vi "Filter_of_Tracks_based_on_areas_differences-2.vi"(4 "error IN":errorcluster, 5 "[IN] Movie Values":T2 {"Particle Fil Setups"."Type of particle filter"."Measurement Parameter" items=["Center of Mass X", "Center of Mass Y", "First Pixel X", "First Pixel Y", "Bounding Rect Left", "Bounding Rect Top", "Bounding Rect Right", "Bounding Rect Bottom", "Max Feret Diameter Start X", "Max Feret Diameter Start Y", "Max Feret Diameter End X", "Max Feret Diameter End Y", "Max Horiz. Segment Length Left", "Max Horiz. Segment Length Right", "Max Horiz. Segment Length Row", "-", "Bounding Rect Width", "Bounding Rect Height", "Bounding Rect Diagonal", "Perimeter", "Convex Hull Perimeter", "Holes' Perimeter", "Max Feret Diameter", "Equivalent Ellipse Major Axis", "Equivalent Ellipse Minor Axis", "Equivalent Ellipse Minor Axis (Feret)", "Equivalent Rect Long Side", "Equivalent Rect Short Side", "Equivalent Rect Diagonal", "Equivalent Rect Short Side (Feret)", "Average Horiz. Segment Length", "Average Vert. Segment Length", "Hydraulic Radius", "Waddel Disk Diameter", "-", "Area", "Holes' Area", "Particle & Holes' Area", "Convex Hull Area", "Image Area", "-", "Number of Holes", "Number of Horiz. Segments", "Number of Vert. Segments", "-", "Orientation", "Max Feret Diameter Orientation", "-", "% Area/Image Area", "% Area/(Particle & Holes' Area)", "Ratio of Equivalent Ellipse Axes", "Ratio of Equivalent Rect Sides", "-", "Elongation Factor", "Compactness Factor", "Heywood Circularity Factor", "Type Factor", "-", "Sum X", "Sum Y", "Sum XX", "Sum XY", "Sum YY", "Sum XXX", "Sum XXY", "Sum XYY", "Sum YYY", "-", "Moment of Inertia XX", "Moment of Inertia XY", "Moment of Inertia YY", "Moment of Inertia XXX", "Moment of Inertia XXY", "Moment of Inertia XYY", "Moment of Inertia YYY", "Norm. Moment of Inertia XX", "Norm. Moment of Inertia XY", "Norm. Moment of Inertia YY", "Norm. Moment of Inertia XXX", "Norm. Moment of Inertia XXY", "Norm. Moment of Inertia XYY", "Norm. Moment of Inertia YYY", "Hu Moment 1", "Hu Moment 2", "Hu Moment 3", "Hu Moment 4", "Hu Moment 5", "Hu Moment 6", "Hu Moment 7"]}, 6 "[IN] Part of mean value (amplitude)\nFor making filtering criteria":dbl, 7 "[IN] Tracks w/t Problems":T3(array[cluster])) -> (0 "error OUT":errorcluster, 2 "[OUT] Oscillating Tracks":cluster{"Short Tracks":dbl[], "Start Pos":i32}[](array[cluster]), 3 "[OUT] Stable Tracks (Filtered)":T3(array[cluster]))   [LabVIEW 2013]
uses:
  <vilib>/Analysis/NI_AALBase.lvlib
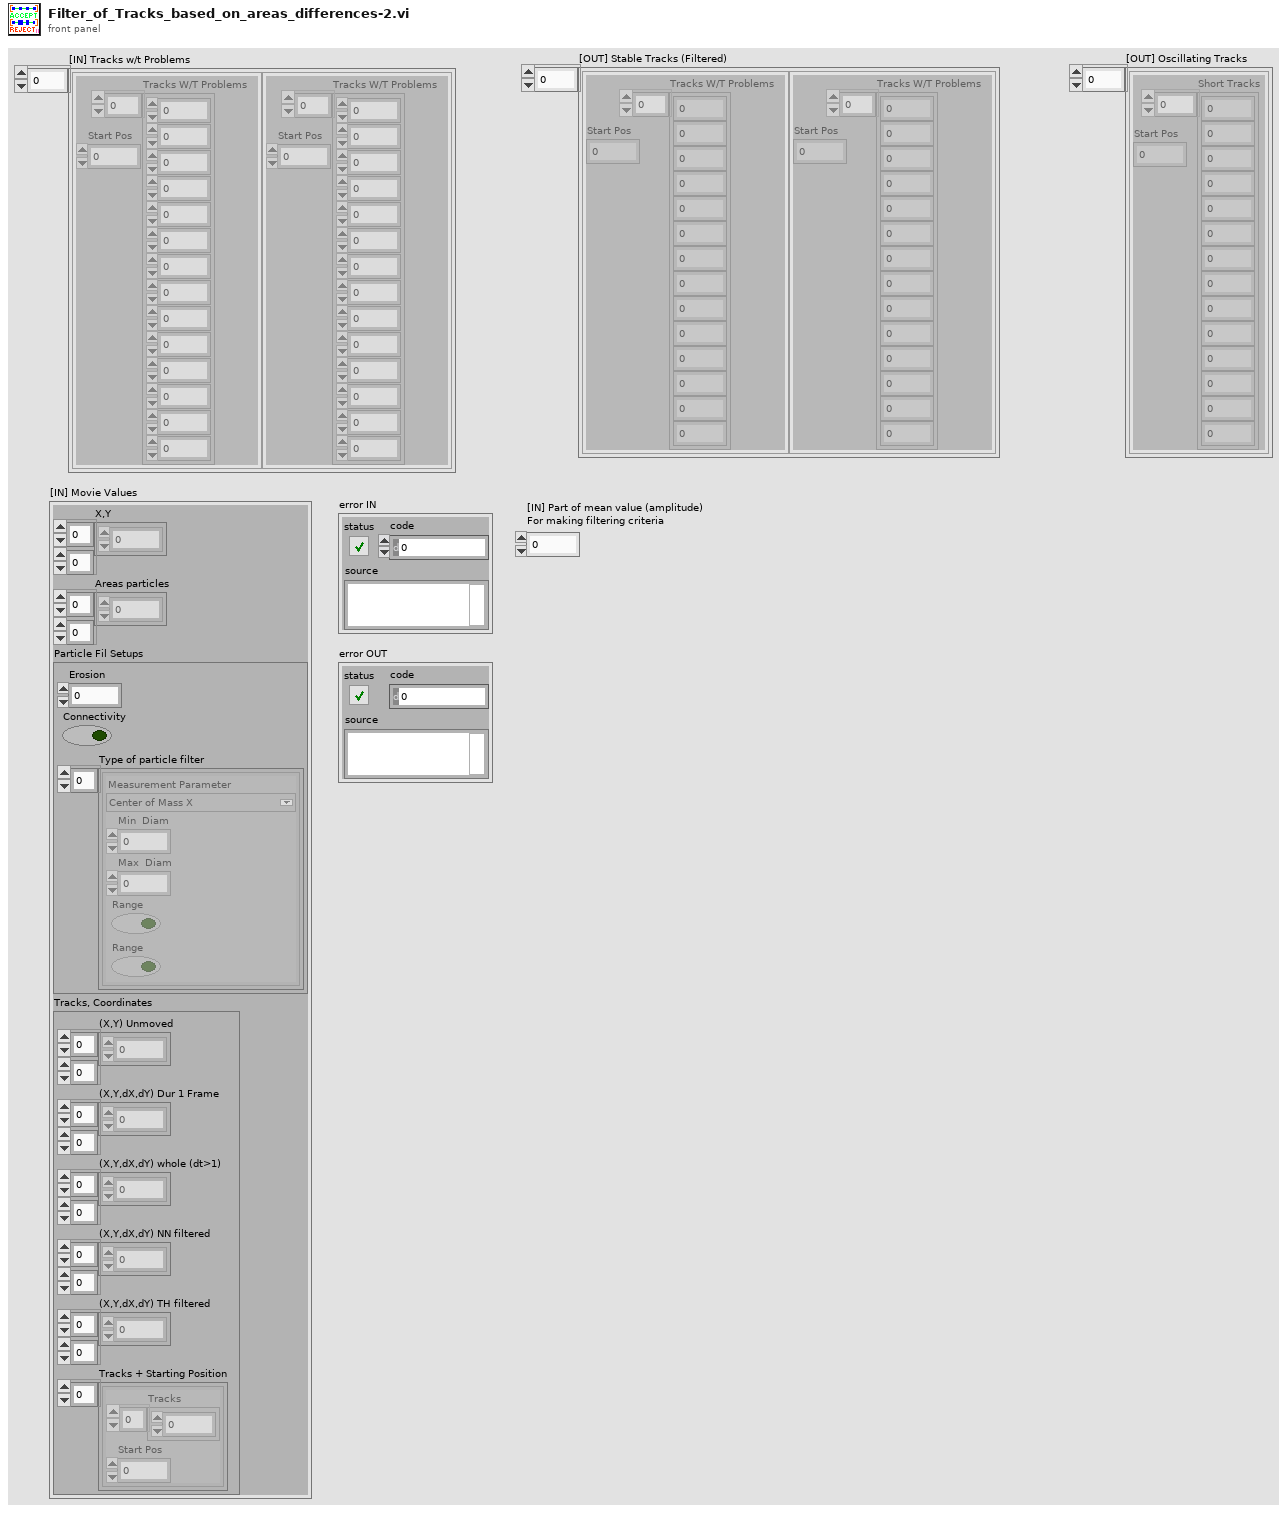
[diagram p1: front panel]
types:
  T1 = typedef "Particle Parameters" = i32
  T2 = cluster{"X,Y":dbl[][], "Areas particles":dbl[][], "Particle Fil Setups":cluster{"Erosion":i32, "Connectivity ":bool, "Type of particle filter":cluster{"Measurement Parameter":T1, "Min  Diam":dbl, "Max  Diam":dbl, "Range":bool, "Range":bool}[]}, "Tracks, Coordinates":cluster{"(X,Y) Unmoved":dbl[][], "(X,Y,dX,dY) Dur 1 Frame":dbl[][], "(X,Y,dX,dY) whole (dt>1)":dbl[][], "(X,Y,dX,dY) NN filtered":dbl[][], "(X,Y,dX,dY) TH filtered":dbl[][], "Tracks + Starting Position":cluster{"Tracks":dbl[], "Start Pos":i32}[]}}
  T3 = cluster{"Tracks W/T Problems":dbl[], "Start Pos":i32}[]
  T4 = cluster{"Oscillating Tracks":dbl[], "Start Pos":i32}
  T5 = cluster{"Oscillating Tracks":dbl[], "Start Pos":i32}[]
  T6 = cluster{"Tracks W/T Problems":dbl[], "Start Pos":i32}
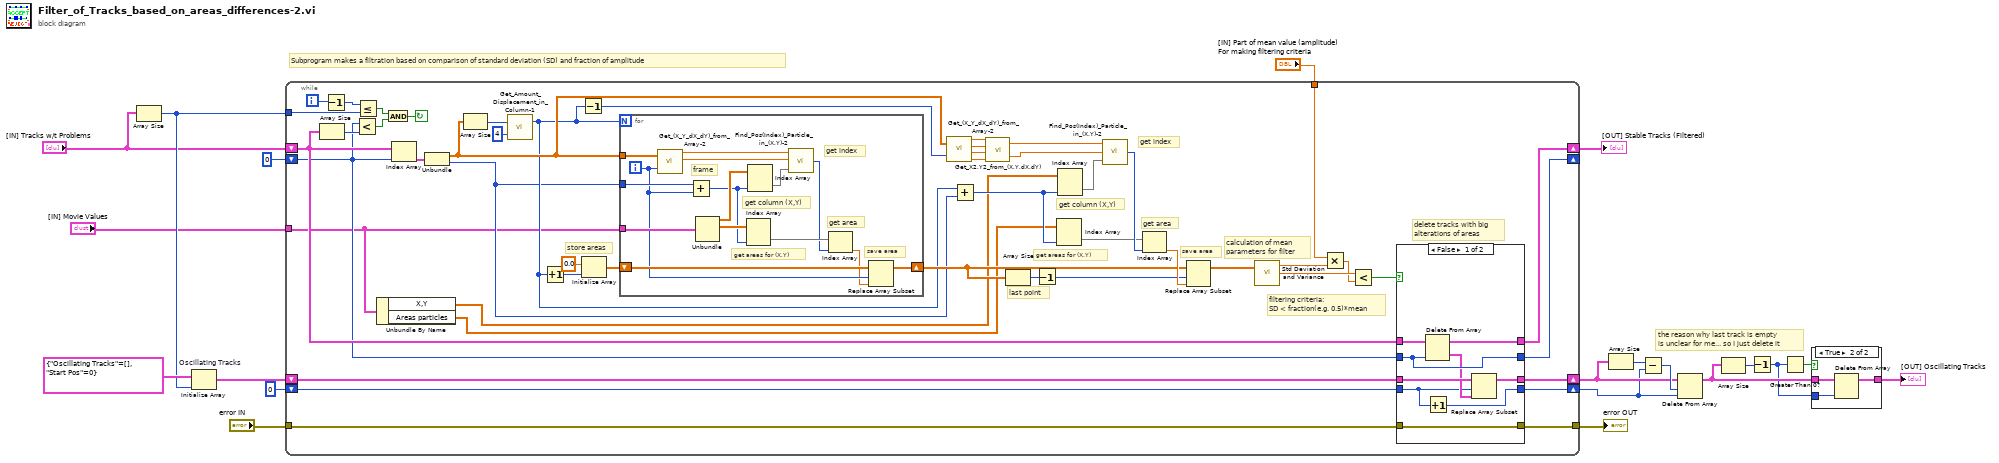
[diagram p0: block diagram]
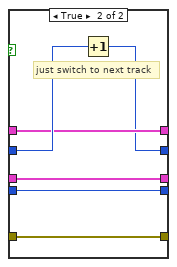
[diagram p3: hidden frame]
diagram:
  # "the reason why last track is empty \nis unclear for me... so I just delete it"
  # "Subprogram makes a filtration based on comparison of standard deviation (SD) and fraction of amplitude"
  n1 = Array Size(array="[IN] Tracks w/t Problems") -> (size(s)=w18:i32)
  n2 = Initialize Array "Oscillating Tracks"(T4 {"Oscillating Tracks"=[], "Start Pos"=0} ("element"), w18) -> (w17:T5)
  n3 = while {
    shift-right: [w58] -> w3
    shift-left: "[IN] Tracks w/t Problems" -> [w60]
    tunnel: w18 -> [w64]
    shift-right: [w57] -> _
    shift-left: 0 -> [w59]
    shift-right: [w54] -> w11
    shift-left: w17 -> [w56]
    shift-right: [w53] -> w10
    shift-left: 0 -> [w55]
    tunnel: "error IN" -> [w52]
    tunnel: [w51] -> w14
    tunnel: "[IN] Movie Values" -> [w23]
    tunnel: "[IN] Part of mean value (amplitude)\nFor making filtering criteria" -> [w46]
    i -> [w65]
    stop <- w66 continue-if-true
    # "last point"
    # "save area"
    # "get area"
    # "get index"
    # "get areas for (X,Y)"
    # "get column (X,Y)"
    # "filtering criteria:\nSD < fraction(e.g. 0.5)*mean"
    # "calculation of mean \nparameters for filter"
    # "store areas"
    # "delete tracks with big\nalterations of areas"
    n4 = Array Size(array=w60) -> (size(s)=w69:i32)
    n5 = Decrement(x=w65) -> (x-1=w67:i32)
    n6 = Less?(x=w59, y=w69) -> (x < y?=w68:bool)
    n7 = Less Or Equal?(x=w67, y=w64) -> (x <= y?=w70:bool)
    n8 = Unbundle By Name(w23) -> ("X,Y"=w22:dbl[][], "Areas particles"=w21:dbl[][])
    n9 = And(x=w70, y=w68) -> (x .and. y?=w66:bool)
    n10 = Index Array(array=w60, index=w59) -> (element=w63:T6)
    n11 = Unbundle(w63) -> ("Tracks W/T Problems"=w32:dbl[], "Start Pos"=w24:i32)
    n12 = Array Size(array=w32) -> (size(s)=w61:i32)
    n13 = call "Get_Amount_Displacement_in_Column-1.vi"("multiplier"=4, "# Rows"=w61) -> ("Displ amount"=w26:i32)  [unwired: 1 out]
    n14 = Increment(x=w26) -> (x+1=w50:i32)
    n15 = Decrement(x=w26) -> (x-1=w27:i32)
    n16 = Initialize Array(0.0 ("Y"), w50) -> (w48:dbl[])
    n17 = for {
      N: w26 -> [_]
      tunnel: w32 -> [w100]
      shift-right: [w93] -> w35
      shift-left: w48 -> [w95]
      tunnel: w23 -> [w97]
      tunnel: w24 -> [w96]
      i -> [w94]
      # "save area"
      # "get area"
      # "get index"
      # "get areas for (X,Y)"
      # "get column (X,Y)"
      # "frame"
      n18 = call "Get_(X_Y_dX_dY)_from_Array-2.vi"("(X,Y,dX,dY)"=w100, "Index of Displacement"=w94) -> ("X"=w99:dbl, "Y"=w98:dbl)  [unwired: 2 out]
      n19 = Add(x=w96, y=w94) -> (x+y=w89:i32)
      n20 = Unbundle(w97) -> ("X,Y"=w92:dbl[][], "Areas particles"=w90:dbl[][])  [unwired: 2 out]
      n21 = Index Array(array=w90, index (col)=w89) -> (element=w88:dbl[])  [unwired: 1 in]
      n22 = Index Array(array=w92, index (col)=w89) -> (element=w91:dbl[])  [unwired: 1 in]
      n23 = call "Find_Pos(Index)_Particle_in_(X,Y)-2.vi"("[X,Y] (n Frame)"=w91, "Y1"=w98, "X1"=w99) -> ("Index in (n) Frame"=w87:i32)
      n24 = Index Array(array=w88, index=w87) -> (element=w86:dbl)
      n25 = Replace Array Subset(array=w95, new element=w86, index=w94) -> (w93:dbl[])
    }
    n26 = call "Get_(X_Y_dX_dY)_from_Array-2.vi"("(X,Y,dX,dY)"=w32, "Index of Displacement"=w27) -> ("X"=w31:dbl, "Y"=w30:dbl, "dX"=w29:dbl, "dY"=w28:dbl)
    n27 = Add(x=w26, y=w24) -> (x+y=w39:i32)
    n28 = call "Get_X2,Y2_from_(X,Y,dX,dY).vi"("dY"=w28, "dX"=w29, "Y1"=w30, "X1"=w31) -> ("Y2 = (Y1+dY)"=w37:dbl, "X2 = (X1+dX)"=w36:dbl)
    n29 = Array Size(array=w35) -> (size(s)=w34:i32)
    n30 = Decrement(x=w34) -> (x-1=w33:i32)
    n31 = Index Array(array=w21, index (col)=w39) -> (element=w40:dbl[])  [unwired: 1 in]
    n32 = Index Array(array=w22, index (col)=w39) -> (element=w38:dbl[])  [unwired: 1 in]
    n33 = call "Find_Pos(Index)_Particle_in_(X,Y)-2.vi"("[X,Y] (n Frame)"=w38, "Y1"=w37, "X1"=w36) -> ("Index in (n) Frame"=w41:i32)
    n34 = Index Array(array=w40, index=w41) -> (element=w42:dbl)
    n35 = Replace Array Subset(array=w35, new element=w42, index=w33) -> (w25:dbl[])
    n36 = call <vilib>:"Std Deviation and Variance.vi"("X"=w25) -> ("mean"=w47:dbl, "standard deviation"=w45:dbl)  [unwired: 1 in, 1 out]
    n37 = Multiply(x=w46, y=w47) -> (x*y=w44:dbl)
    n38 = Less?(x=w45, y=w44) -> (x < y?=w43:bool)
    n39 = case shown="False" w43 {
      tunnel: w60 -> [w79 w84]
      tunnel: w59 -> [w77 w85]
      tunnel: [w78 w84] -> w58
      tunnel: [w77 w83] -> w57
      tunnel: w56 -> [w76 w82]
      tunnel: w55 -> [w73 w81]
      tunnel: [w74 w82] -> w54
      tunnel: [w72 w81] -> w53
      tunnel: w52 -> [w71 w80]
      tunnel: [w71 w80] -> w51
      frame False {
        n40 = Delete From Array(array=w79, index=w77) -> (deleted portion=w75:T6, array with subset deleted=w78:T3)  [unwired: 1 in]
        n41 = Increment(x=w73) -> (x+1=w72:i32)
        n42 = Replace Array Subset(array=w76, new element=w75, index=w73) -> (w74:T5)
      }
      frame True {
        # "just switch to next track"
        n43 = Increment(x=w85) -> (x+1=w83:i32)
      }
    }
  }
  "[OUT] Stable Tracks (Filtered)" <- w3
  "error OUT" <- w14
  n44 = Array Size(array=w11) -> (size(s)=w13:i32)
  n45 = Subtract(x=w13, y=w10) -> (x-y=w12:i32)
  n46 = Delete From Array(array=w11, length=w12, index=w10) -> (array with subset deleted=w9:T5)  [unwired: 1 out]
  n47 = Array Size(array=w9) -> (size(s)=w8:i32)
  n48 = Decrement(x=w8) -> (x-1=w6:i32)
  n49 = Greater Than 0?(x=w6) -> (x > 0?=w5:bool)
  n50 = case shown="True" w5 {
    tunnel: w9 -> [w101 w104]
    tunnel: [w101 w103] -> w7
    tunnel: w6 -> [_ w102]
    frame False {
    }
    frame True {
      n51 = Delete From Array(array=w104, index=w102) -> (array with subset deleted=w103:T5)  [unwired: 1 in, 1 out]
    }
  }
  "[OUT] Oscillating Tracks" <- w7
